vi "solar_voy Write IDOffset.vi"(8 "error in (no error)":errorcluster, 9 "ID Offset":u16, 10 "Target Name":string, 11 "Voyager Refnum in":T1) -> (0 "error out":errorcluster, 3 "Voyager Refnum out":T1)   [LabVIEW 2018]
doc: "Writes the voyager id for a specific target into the voyager queue."
uses:
  solar_voy_ctl Voyager Refnum.ctl
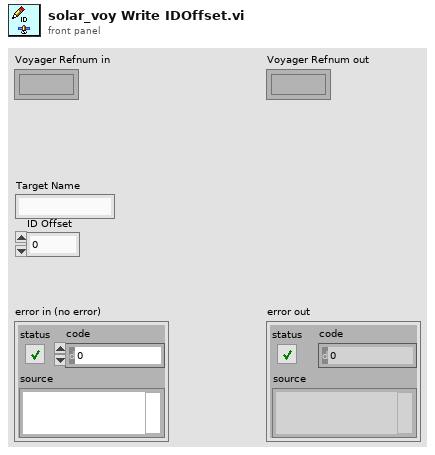
[diagram p1: front panel]
types:
  T1 = typedef "solar_voy_ctl Voyager Refnum.ctl" = refnum<k1>
  T2 = typedef "solar_voy_ctl Voyager.ctl" = cluster{"PACKETS":T3[], "COSMOS_Root":path, "CMD_HDR":T8, "TLM_HDR":T8, "TCPs":T9[], "VoyagerIDOffset":cluster{"VoyagerIDOffset":u16[], "Target Names":string[]}}
  T3 = typedef "solar_voy_def_ctl PACKET.ctl" = cluster{"PACKET_ID":T4, "ENDIAN":enum8{"BIG", "LITTLE"}, "DESC":string, "HZRD":bool, "ITEMS":T5[], "NoExport":bool, "last_time":timestamp, "last_count":u32, "last_data":string}
  T4 = typedef "solar_voy_def_ctl PACKET_ID.ctl" = cluster{"ID":u16, "CMD":enum8{"CMD", "TLM"}, "TARGET":string, "PACKET":string}
  T5 = typedef "solar_voy_def_ctl ITEM.ctl" = cluster{"NAME":string, "OFFSET":i32, "SIZE":i32, "TYPE":T6, "EACH_SIZE":i32, "LVTYPE":T7, "MIN":dbl, "MAX":dbl, "DEFAULT":string, "DESC":string, "ID":bool, "MODIFIERS":variant, "last_value":variant}
  T6 = typedef "solar_voy_def_ctl ITEM TYPE.ctl" = enum8{"BLOCK", "INT", "UINT", "FLOAT", "STRING"}
  T7 = typedef "solar_type Item Type.ctl" = enum16{"NULL", "UNKNOWN", "CLUSTER", "I8", "I16", "I32", "I64", "U8", "U16", "U32", "U64", "U8_ENUM", "U16_ENUM", "U32_ENUM", "SGL", "DBL", "BOOLEAN", "STRING", "PATH", "VISA", "TAG", "TIME", "I8_1D", "I16_1D", "I32_1D", "I64_1D", "U8_1D", "U16_1D", "U32_1D", "U64_1D", "U8_ENUM_1D", "U16_ENUM_1D", "U32_ENUM_1D", "SGL_1D", "DBL_1D", "BOOLEAN_1D", "STRING_1D", "PATH_1D", "VISA_1D", "TAG_1D", "TIME_1D", "I8_2D", "I16_2D", "I32_2D", "I64_2D", "U8_2D", "U16_2D", "U32_2D", "U64_2D", "U8_ENUM_2D", "U16_ENUM_2D", "U32_ENUM_2D", "SGL_2D", "DBL_2D", "BOOLEAN_2D", "STRING_2D", "PATH_2D", "VISA_2D", "TAG_2D", "TIME_2D"}
  T8 = typedef "solar_voy_def_ctl HDR.ctl" = cluster{"ITEMS":T5[], "LENGTH_NAME":string, "LENGTH_VALUE_OFFSET":i32, "ID_NAME":string, "ENDIAN":enum8{"BIG", "LITTLE"}, "GUID_NAME":string, "DEFAULT_TARGET":string, "DEFAULT_PACKET":string, "DEFAULT_ERROR":string}
  T9 = typedef "solar_voy_ctl TCP.ctl" = cluster{"Connected":bool, "Port":u16, "Listener":refnum<k5>, "ServerIP":string, "TCP":refnum<k5>, "Setup":T10, "VIRefnum":refnum<vi>, "TARGETS_CMD":string[], "TARGETS_TLM":string[]}
  T10 = typedef "solar_voy_ctl Port Setup.ctl" = enum8{"SERVER", "CLIENT", "SERVER_CMD", "SERVER_TLM"}
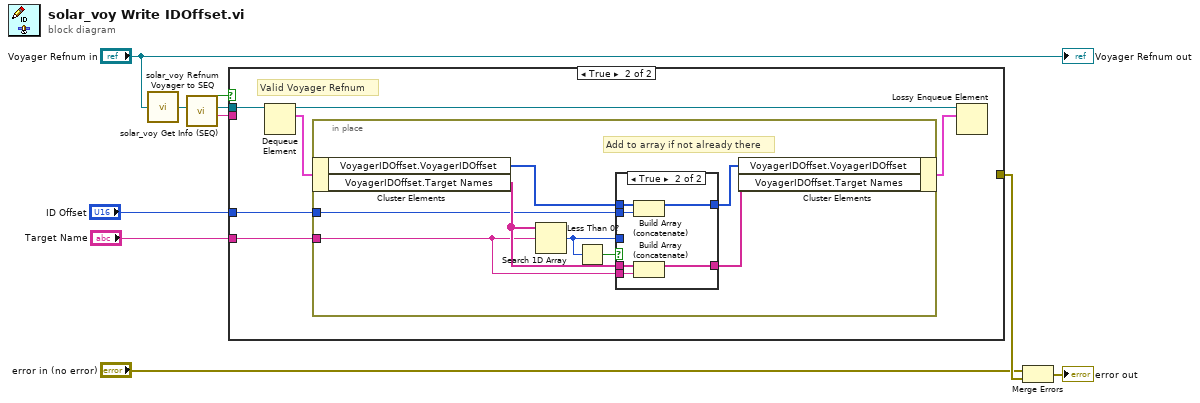
[diagram p0: block diagram]
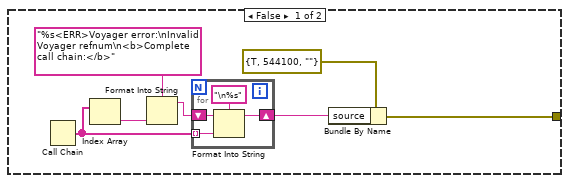
[diagram p2: hidden frame]
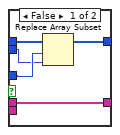
[diagram p3: hidden frame]
diagram:
  n1 = call "solar_voy Refnum Voyager to SEQ.vi"("Voyager Refnum"="Voyager Refnum in") -> ("Voyager SEQ"=w10:refnum<queue>)
  n2 = call "solar_voy Get Info (SEQ).vi"("Voyager SEQ in"=w10) -> ("Interface Name"=w8:string, "Voyager SEQ out"=w9:refnum<queue>, "Valid?"=w7:bool)  [unwired: 8 in]
  n3 = case shown="True" w7 {
    tunnel: w9 -> [_ w27]
    tunnel: w8 -> [_ _]
    tunnel: [w11 _] -> w6
    tunnel: "Target Name" -> [_ w23]
    tunnel: "ID Offset" -> [_ w22]
    frame False {
      n4 = Call Chain() -> (call chain=w14:string[])
      n5 = Index Array(array=w14) -> (element=w16:string)  [unwired: 1 in]
      n6 = Format Into String(format string="%s<ERR>Voyager error:\nInvalid Voyager refnum\n<b>Complete call chain:</b>", w16) -> (resulting string=w15:string)  [unwired: 2 in, 1 out]
      n7 = for {
        tunnel: w14 -> [w21] mode=indexing
        shift-right: [w20] -> w13
        shift-left: w15 -> [w19]
        n8 = Format Into String(format string="\n%s", initial string=w19, w21) -> (resulting string=w20:string)  [unwired: 1 in, 1 out]
      }
      n9 = Bundle By Name(cluster=errorcluster {"status"=TRUE, "code"=544100, "source"=""} ("error in (no error)"), "source"=w13) -> (w11:errorcluster)
    }
    frame True {
      # "Valid Voyager Refnum"
      n10 = Dequeue Element(queue=w27) -> (queue out=w24:refnum<queue>, element=w26:T2)  [unwired: 2 in, 2 out]
      n11 = in-place {
        in-place-border: w23 -> [w33]
        in-place-border: w22 -> [w31]
        # "Add to array if not already there"
        n12 = in-place-cluster #1(w26) -> ("VoyagerIDOffset.VoyagerIDOffset"=w30:u16[], "VoyagerIDOffset.Target Names"=w34:string[])
        n13 = Search 1D Array(1D array=w34, element=w33) -> (index of element=w28:i32)  [unwired: 1 in]
        n14 = Less Than 0?(x=w28) -> (x < 0?=w35:bool)
        n15 = case shown="True" w35 {
          tunnel: w34 -> [w36 w46]
          tunnel: w33 -> [_ w45]
          tunnel: [w36 w44] -> w32
          tunnel: w30 -> [w40 w43]
          tunnel: w31 -> [w38 w42]
          tunnel: [w37 w41] -> w29
          tunnel: w28 -> [w39 _]
          frame False {
            n16 = Replace Array Subset(array=w40, new element=w38, index=w39) -> (w37:u16[])
          }
          frame True {
            n17 = Build Array (concatenate)(w43, w42) -> (w41:u16[])
            n18 = Build Array (concatenate)(w46, w45) -> (w44:string[])
          }
        }
        n19 = in-place-cluster #1("VoyagerIDOffset.VoyagerIDOffset"=w29, "VoyagerIDOffset.Target Names"=w32) -> (w25:T2)
      }
      n20 = Lossy Enqueue Element(queue=w24, element=w25) -> ()  [unwired: 1 in, 4 out]
    }
  }
  n21 = Merge Errors("error in (no error)", w6) -> (→"error out":errorcluster)
  "Voyager Refnum out" <- "Voyager Refnum in"
